vi "SQL查询.vi"(7 "condition":string, 8 "error in (no error)":errorcluster, 9 "columns":string[](array[string]), 10 "table输入":string(combo), 11 "database":string(combo)) -> (0 "error out":errorcluster, 1 "拆分数据":bool, 2 "columns输出":string[](array[string]), 3 "data":string[][](table))   [LabVIEW 2016, in "数据传输系统-04.lvlib"]
uses:
  <vilib>/Utility/sysdir.llb/System Directory Type.ctl
  <vilib>/addons/database/Connection.llb/DB Tools Open Connec (String).vi
  <vilib>/addons/database/_DB Variant To Data/Database Variant To Data.xnode
  <vilib>/addons/database/NI_Database_API.lvlib
panel:
  out "元素":string
  out "子数组":string[](array[string])
  # "时间 > #2021/01/15 08:00:00#and 时间 < #2021/04/15 08:00:00# order by 时间 asc"
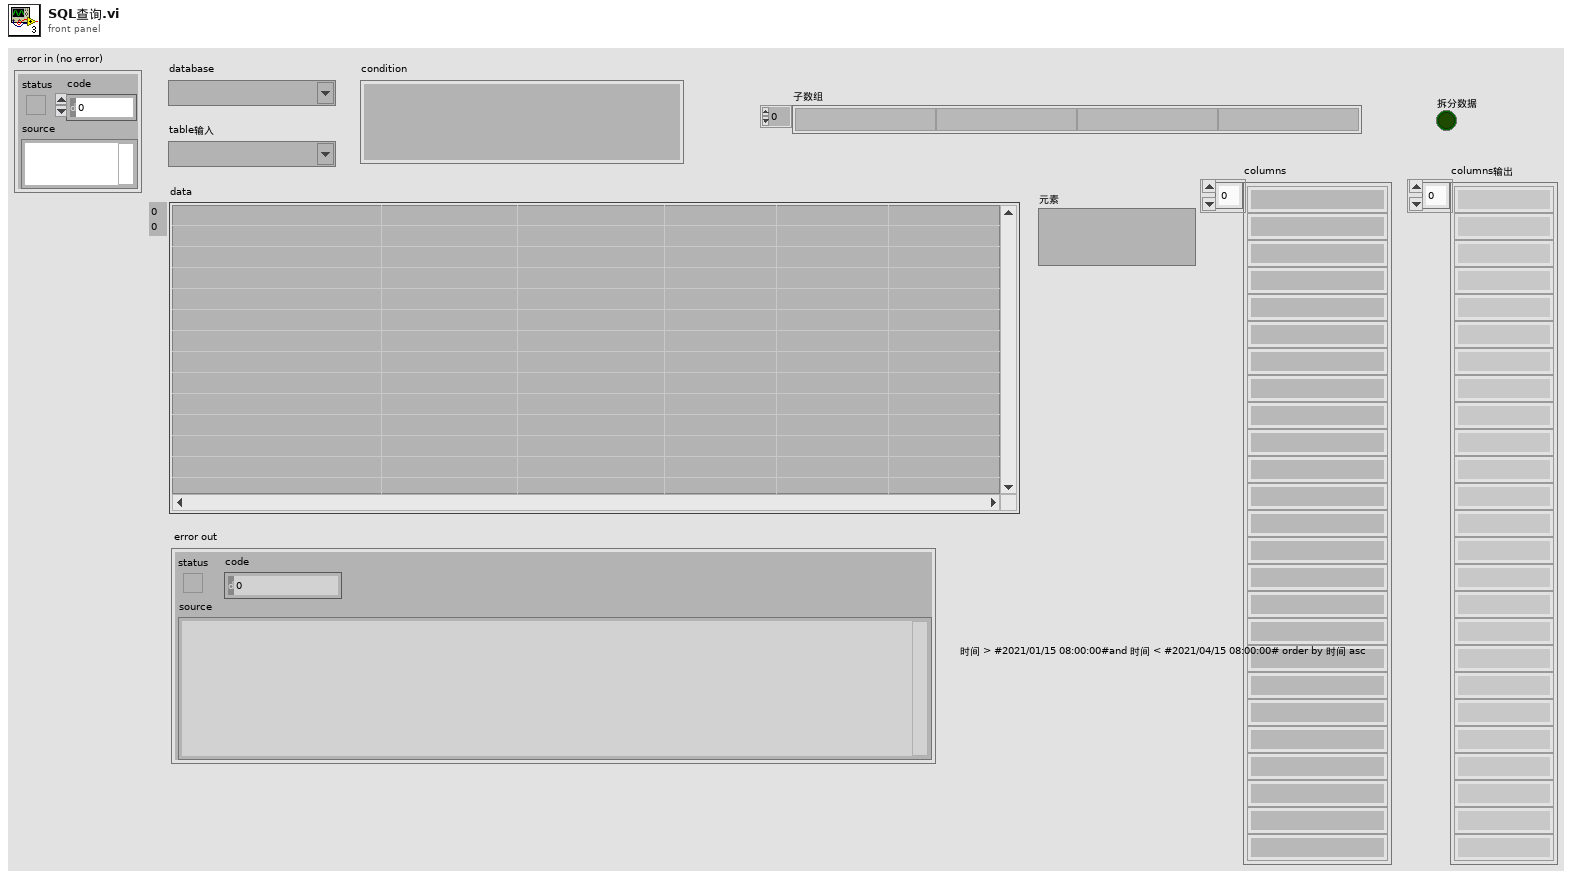
[diagram p1: front panel]
types:
  T1 = typedef "System Directory Type.ctl" = i32
  T2 = typedef "NI_Database_API.lvlib/Conn ObjectReference.ctl" = refnum<k1>
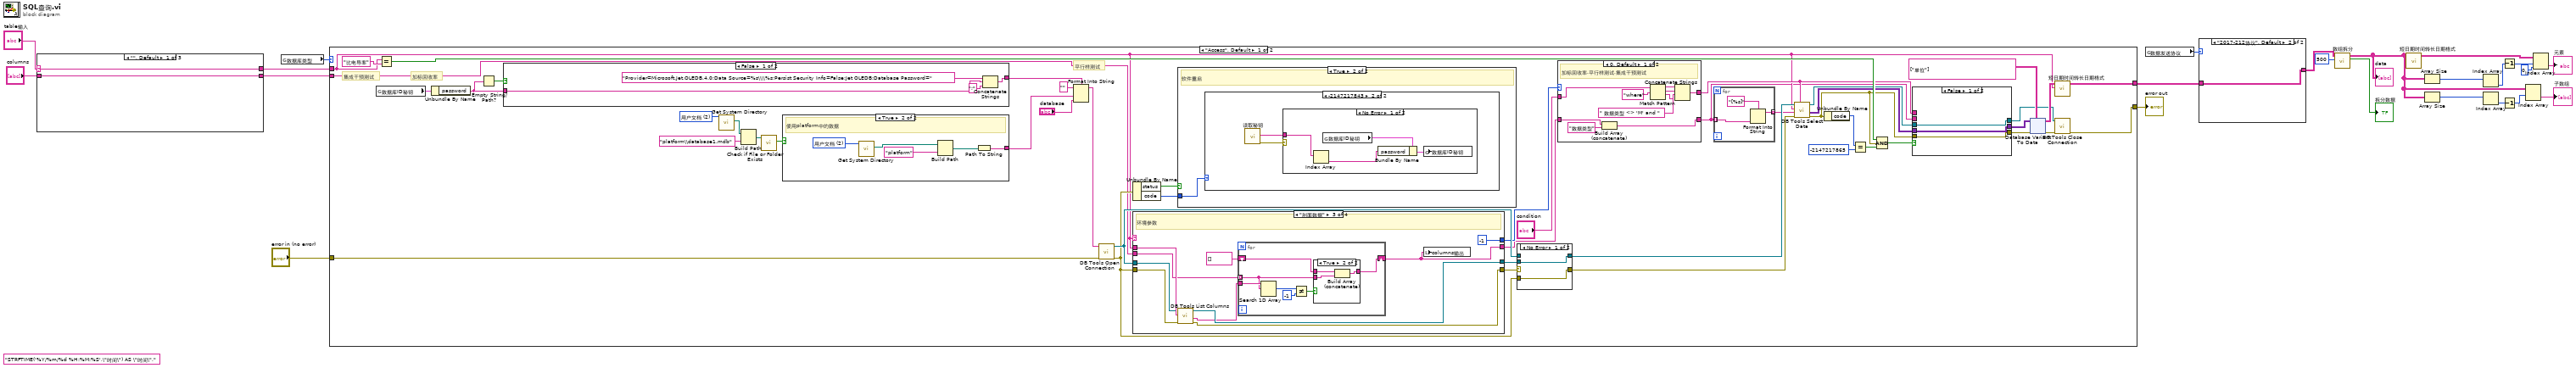
[diagram p0: block diagram]
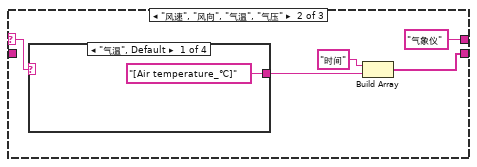
[diagram p2: hidden frame]
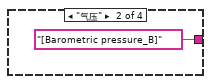
[diagram p3: hidden frame]
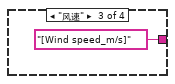
[diagram p4: hidden frame]
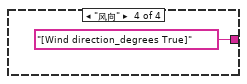
[diagram p5: hidden frame]
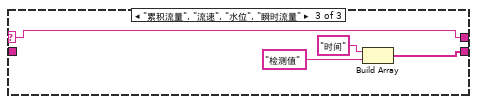
[diagram p6: hidden frame]
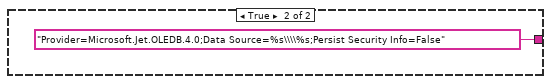
[diagram p7: hidden frame]
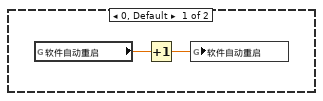
[diagram p9: hidden frame]
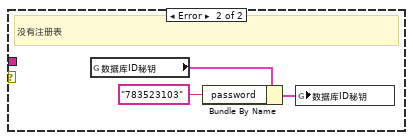
[diagram p10: hidden frame]
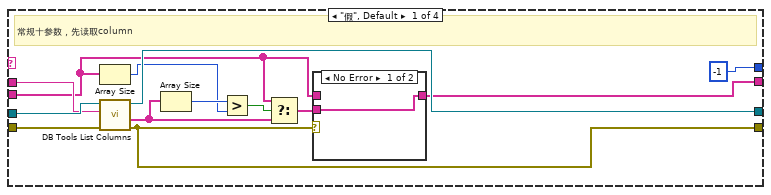
[diagram p13: hidden frame]
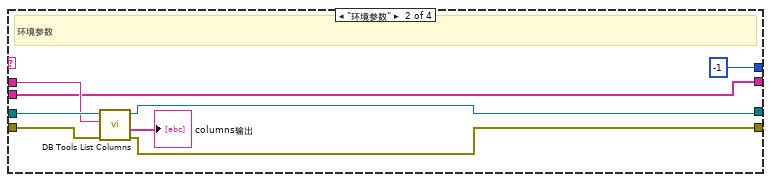
[diagram p15: hidden frame]
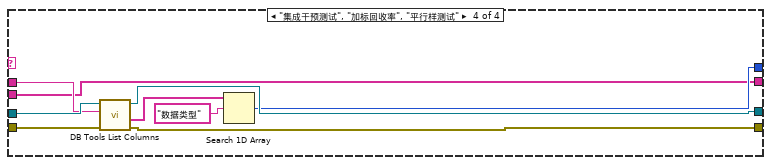
[diagram p17: hidden frame]
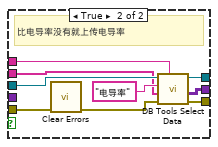
[diagram p18: hidden frame]
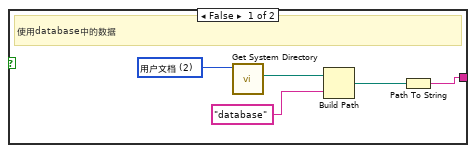
[diagram p19: hidden frame]
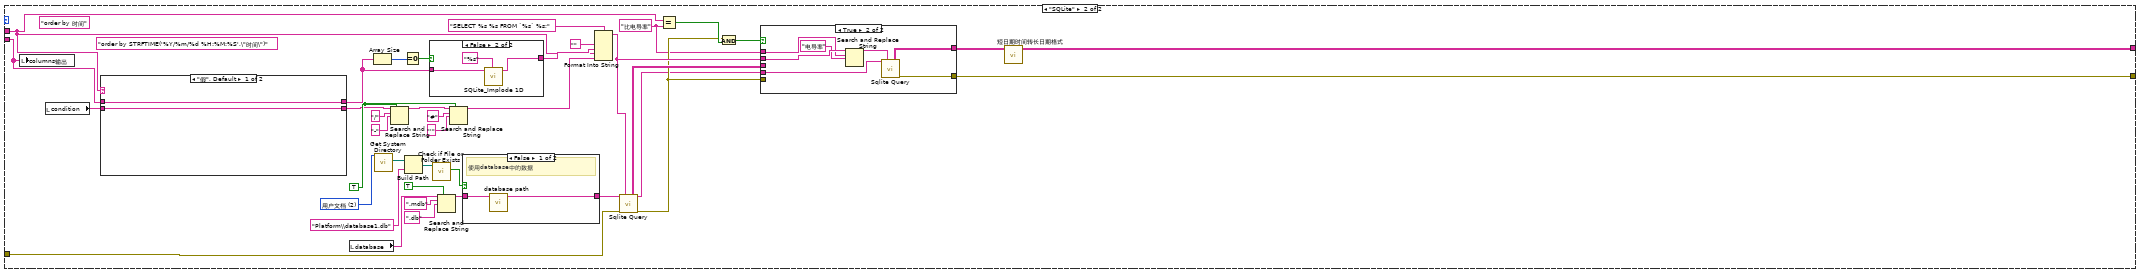
[diagram p20: hidden frame]
diagram:
  (unwired) "STRFTIME('%Y/%m/%d %H:%M:%S',\"时间\") AS \"时间\"," ("输入 1")
  n1 = case shown="\"\", Default" "table输入" {
    selector: "table输入" -> [w25 w29 w35]
    tunnel: [w25 "气象仪" w35] -> w4
    tunnel: "columns" -> [w24 _ _]
    tunnel: [w24 w26 w37] -> w5
    frame "", Default {
    }
    frame "风速", "风向", "气温", "气压" {
      n2 = case shown="\"气温\", Default" w29 {
        tunnel: ["[Air temperature_℃]" "[Barometric pressure_B]" "[Wind speed_m/s]" "[Wind direction_degrees True]"] -> w27
        frame "气温", Default {
        }
        frame "气压" {
        }
        frame "风速" {
        }
        frame "风向" {
        }
      }
      n3 = Build Array("时间", w27) -> (w26:string[])
    }
    frame "累积流量", "流速", "水位", "瞬时流量" {
      n4 = Build Array("时间", "检测值") -> (w37:string[])
    }
  }
  n5 = global read "断电保存全局.vi" "数据库类型"() -> (w8:enum16{"Access", "SQLite"})
  n6 = case shown="\"Access\", Default" w8 {
    tunnel: [w80 w274] -> w23
    tunnel: [w52 w250] -> w11
    tunnel: "error in (no error)" -> [w45 w243]
    tunnel: w5 -> [w43 w246]
    tunnel: w4 -> [w42 w245]
    frame "Access", Default {
      w78 = T1 2 items=["用户目录"=0, "用户桌面"=1, "用户文档"=2, "用户应用程序数据"=3, "用户设置"=4, "用户临时目录"=5, "公共文档"=6, "公共应用程序数据"=7, "公共设置"=8, "公共缓存"=13, "系统核心库"=9, "系统安装库"=10, "应用程序文件"=11, "启动盘根目录"=12] ("system directory type")
      # "集成干预测试"
      # "平行样测试"
      # "加标回收率"
      n7 = global read "外部交互全局.vi" "数据库ID秘钥"() -> (w46:cluster{"userID":string, "password":string})
      n8 = Equal?(x=w42, y="比电导率") -> (x = y?=w72:bool)
      n9 = Unbundle By Name(w46) -> ("password"=w47:string)
      n10 = Empty String/Path?(string/path=w47) -> (empty?=w49:bool)
      n11 = case shown="False" w49 {
        tunnel: [w89 "Provider=Microsoft.Jet.OLEDB.4.0;Data Source=%s\\\\%s;Persist Security Info=False" ("格式字符串")] -> w48
        tunnel: w47 -> [w92 _]
        frame False {
          n12 = Concatenate Strings("Provider=Microsoft.Jet.OLEDB.4.0;Data Source=%s\\\\%s;Persist Security Info=False;Jet OLEDB:Database Password=" ("格式字符串"), w92, ";" ("字符串")) -> (w89:string)
        }
        frame True {
        }
      }
      n13 = call <vilib>:"Get System Directory.vi"("system directory type"=w78) -> ("system directory"=w79:path)  [unwired: 10 in]
      n14 = Build Path(base path=w79, name or relative path="platform\\database1.mdb" ("condition")) -> (appended path=w77:path)
      n15 = call <vilib>:"Check if File or Folder Exists.vi"("path"=w77) -> ("file or folder exists?"=w75:bool)  [unwired: 8 in, 2 out]
      n16 = case shown="True" w75 {
        tunnel: [w187 w192] -> w74
        frame False {
          w190 = T1 2 items=["用户目录"=0, "用户桌面"=1, "用户文档"=2, "用户应用程序数据"=3, "用户设置"=4, "用户临时目录"=5, "公共文档"=6, "公共应用程序数据"=7, "公共设置"=8, "公共缓存"=13, "系统核心库"=9, "系统安装库"=10, "应用程序文件"=11, "启动盘根目录"=12] ("system directory type")
          # "使用database中的数据"
          n17 = call <vilib>:"Get System Directory.vi"("system directory type"=w190) -> ("system directory"=w189:path)  [unwired: 10 in]
          n18 = Build Path(base path=w189, name or relative path="database" ("condition")) -> (appended path=w191:path)
          n19 = Path To String(path=w191) -> (string=w187:string)
        }
        frame True {
          w196 = T1 2 items=["用户目录"=0, "用户桌面"=1, "用户文档"=2, "用户应用程序数据"=3, "用户设置"=4, "用户临时目录"=5, "公共文档"=6, "公共应用程序数据"=7, "公共设置"=8, "公共缓存"=13, "系统核心库"=9, "系统安装库"=10, "应用程序文件"=11, "启动盘根目录"=12] ("system directory type")
          # "使用platform中的数据"
          n20 = call <vilib>:"Get System Directory.vi"("system directory type"=w196) -> ("system directory"=w195:path)  [unwired: 10 in]
          n21 = Build Path(base path=w195, name or relative path="platform" ("condition")) -> (appended path=w193:path)
          n22 = Path To String(path=w193) -> (string=w192:string)
        }
      }
      n23 = Format Into String(format string=w48, initial string="" ("初始字符串"), w74, "database") -> (resulting string=w82:string)  [unwired: 1 in, 1 out]
      n24 = call-poly <vilib>:"DB Tools Open Connection.vi"("error in (no error)"=w45, "connection information"=w82) -> ("error out"=w53:errorcluster, "connection reference"=w58:T2)  [unwired: 6 in]
      n25 = Unbundle By Name(w53) -> ("status"=w51:bool, "code"=w41:i32)
      n26 = case shown="\"剖面数据\"" w42 {
        tunnel: w58 -> [w133 w144 w152 w174]
        tunnel: w53 -> [w130 w143 w151 w172]
        tunnel: [w131 w142 w149 w171] -> w60
        tunnel: [w125 w141 w150 w170] -> w61
        tunnel: w42 -> [w132 w140 w153 w173]
        tunnel: [-1 ("index of element") -1 ("index of element") -1 ("index of element") w167] -> w56
        tunnel: w43 -> [w122 w137 w148 w166]
        tunnel: [w123 w137 w145 w166] -> w54
        frame "假", Default {
          # "常规十参数，先读取column"
          n27 = Array Size(array=w122) -> (size(s)=w127:i32)
          n28 = call <vilib>:"DB Tools List Columns.vi"("error in (no error)"=w130, "table"=w132, "connection reference"=w133) -> ("error out"=w125:errorcluster, "columns"=w126:string[], "connection reference out"=w131:T2)  [unwired: 1 in, 1 out]
          n29 = Array Size(array=w126) -> (size(s)=w128:i32)
          n30 = Greater?(x=w128, y=w127) -> (0:w129:bool)
          n31 = Select(t=w122, s=w129, f=w126) -> (s? t:f=w124:string[])
          n32 = case shown="No Error" w125 {
            tunnel: w124 -> [w135 _]
            tunnel: [w135 w136] -> w123
            tunnel: w122 -> [_ w136]
            frame No Error {
            }
            frame Error {
            }
          }
        }
        frame "环境参数" {
          # "环境参数"
          n33 = call <vilib>:"DB Tools List Columns.vi"("error in (no error)"=w143, "table"=w140, "connection reference"=w144) -> ("error out"=w141:errorcluster, "columns"=→"columns输出":string[], "connection reference out"=w142:T2)  [unwired: 1 in, 1 out]
        }
        frame "剖面数据" {
          # "环境参数"
          n34 = call <vilib>:"DB Tools List Columns.vi"("error in (no error)"=w151, "table"=w153, "connection reference"=w152) -> ("error out"=w150:errorcluster, "columns"=w147:string[], "connection reference out"=w149:T2)  [unwired: 1 in, 1 out]
          n35 = for {
            tunnel: w148 -> [w157] mode=indexing
            tunnel: w147 -> [w161]
            shift-right: [w155] -> w145
            shift-left: string[] [] -> [w158]
            n36 = Search 1D Array(1D array=w161, element=w157) -> (index of element=w160:i32)  [unwired: 1 in]
            n37 = Not Equal?(x=w160, y=-1) -> (x != y?=w156:bool)
            n38 = case shown="True" w156 {
              tunnel: w158 -> [w162 w165]
              tunnel: w157 -> [_ w164]
              tunnel: [w162 w163] -> w155
              frame False {
              }
              frame True {
                n39 = Build Array (concatenate)(w165, w164) -> (w163:string[])
              }
            }
          }
          n40 = local write "columns输出"(w145) -> ()
        }
        frame "集成干预测试", "加标回收率", "平行样测试" {
          n41 = call <vilib>:"DB Tools List Columns.vi"("error in (no error)"=w172, "table"=w173, "connection reference"=w174) -> ("error out"=w170:errorcluster, "columns"=w169:string[], "connection reference out"=w171:T2)  [unwired: 1 in, 1 out]
          n42 = Search 1D Array(1D array=w169, element="数据类型" ("元素")) -> (index of element=w167:i32)  [unwired: 1 in]
        }
      }
      n43 = case shown="True" w51 {
        tunnel: w41 -> [_ w94]
        frame False {
        }
        frame True {
          # "软件重启"
          n44 = case shown="-2147217843" w94 {
            frame 0, Default {
              n45 = global read "全局1.vi" "软件自动重启"() -> (w96:dbl)
              n46 = Increment(x=w96) -> (x+1=w95:dbl)
              n47 = global write "全局1.vi" "软件自动重启"(w95) -> ()
            }
            frame -2147217843 {
              n48 = call "读取秘钥.vi"() -> ("error out"=w97:errorcluster, "值"=w98:string[])  [unwired: 9 in, 1 out]
              n49 = case shown="No Error" w97 {
                tunnel: w98 -> [w102 _]
                frame No Error {
                  n50 = Index Array(array=w102) -> (element=w99:string)  [unwired: 1 in]
                  n51 = global read "外部交互全局.vi" "数据库ID秘钥"() -> (w100:cluster{"userID":string, "password":string})
                  n52 = Bundle By Name(cluster=w100, "password"=w99) -> (w101:cluster{"userID":string, "password":string})
                  n53 = global write "外部交互全局.vi" "数据库ID秘钥"(w101) -> ()
                }
                frame Error {
                  # "没有注册表"
                  n54 = global read "外部交互全局.vi" "数据库ID秘钥"() -> (w104:cluster{"userID":string, "password":string})
                  n55 = Bundle By Name(cluster=w104, "password"="783523103") -> (w105:cluster{"userID":string, "password":string})
                  n56 = global write "外部交互全局.vi" "数据库ID秘钥"(w105) -> ()
                }
              }
            }
          }
        }
      }
      n57 = case shown="No Error" w61 {
        selector: w61 -> [_ w121]
        tunnel: w60 -> [w119 _]
        tunnel: [w119 w120] -> w59
        tunnel: w58 -> [_ w120]
        tunnel: [w118 w121] -> w57
        tunnel: w53 -> [w118 _]
        frame No Error {
        }
        frame Error {
        }
      }
      n58 = case "条件结构" shown="0, Default" w56 {
        tunnel: "condition" -> [w113 w116]
        tunnel: w54 -> [w115 w117]
        tunnel: [w107 w117] -> w40
        tunnel: [w106 w116] -> w50
        frame 0, Default {
          # "加标回收率,平行样测试,集成干预测试"
          n59 = Build Array (concatenate)(w115, "数据类型" ("元素")) -> (w107:string[])
          n60 = Match Pattern(string=w113, regular expression="where" ("正则表达式")) -> (before substring=w111:string, match substring=w110:string, after substring=w108:string)  [unwired: 1 in, 1 out]
          n61 = Concatenate Strings(w111, w110, " 数据类型 <> 'M' and " ("字符串"), w108) -> (w106:string)
        }
        frame -1 {
        }
      }
      n62 = for {
        tunnel: w40 -> [w88] mode=indexing
        tunnel: [w87] -> w39 mode=indexing
        n63 = Format Into String(format string="[%s]" ("格式字符串"), w88) -> (resulting string=w87:string)  [unwired: 2 in, 1 out]
      }
      n64 = call <vilib>:"DB Tools Select Data.vi"("condition"=w50, "error in (no error)"=w57, "columns"=w39, "table"=w42, "connection reference"=w59) -> ("error out"=w65:errorcluster, "data"=w67:variant[][], "connection reference out"=w70:T2)  [unwired: 1 in]
      n65 = Unbundle By Name(w65) -> ("code"=w64:i32)
      n66 = Equal?(x=w64, y=-2147217865 ("code")) -> (x = y?=w62:bool)
      n67 = Compound Arithmetic op=AND ("复合运算")(w72, w65, w62) -> (w71:bool)
      n68 = case shown="False" w71 {
        tunnel: w50 -> [_ w186]
        tunnel: w70 -> [w177 w185]
        tunnel: [w177 w180] -> w69
        tunnel: [w176 w181] -> w68
        tunnel: w67 -> [w176 _]
        tunnel: w65 -> [w175 w183]
        tunnel: [w175 w179] -> w66
        tunnel: w40 -> [_ w178]
        frame False {
        }
        frame True {
          # "比电导率没有就上传电导率"
          n69 = call <vilib>:"Clear Errors.vi"("error in (no error)"=w183) -> ("error out"=w182:errorcluster)  [unwired: 5 in, 1 out]
          n70 = call <vilib>:"DB Tools Select Data.vi"("condition"=w186, "error in (no error)"=w182, "columns"=w178, "table"="电导率", "connection reference"=w185) -> ("error out"=w179:errorcluster, "data"=w181:variant[][], "connection reference out"=w180:T2)  [unwired: 1 in]
        }
      }
      n71 = xnode "Database Variant To Data"("database variant"=w68, "error in (no error)"=w66, "type"=string[][] [["单位"]]) -> ("data"=w81:string[][], "error out"=w83:errorcluster)
      n72 = call "短日期时间转长日期格式.vi"("table输入"=w42, "data"=w81) -> ("输出数组"=w80:string[][])  [unwired: 9 in]
      n73 = call <vilib>:"DB Tools Close Connection.vi"("error in (no error)"=w83, "connection reference"=w69) -> ("error out"=w52:errorcluster)  [unwired: 5 in]
    }
    frame "SQLite" {
      w248 = "比电导率" ("y")
      (unwired) "order by STRFTIME('%Y/%m/%d %H:%M:%S',\"时间\")" ("替换字符串(\"\")")
      (unwired) "order by 时间" ("搜索字符串")
      w259 = TRUE ("替换全部？(F)")
      w276 = T1 2 items=["用户目录"=0, "用户桌面"=1, "用户文档"=2, "用户应用程序数据"=3, "用户设置"=4, "用户临时目录"=5, "公共文档"=6, "公共应用程序数据"=7, "公共设置"=8, "公共缓存"=13, "系统核心库"=9, "系统安装库"=10, "应用程序文件"=11, "启动盘根目录"=12] ("system directory type")
      n74 = local write "columns输出"(w246) -> ()
      n75 = local read "condition"() -> (w258:string)
      n76 = case shown="\"假\", Default" w245 {
        tunnel: w258 -> [w290 w296]
        tunnel: w246 -> [w289 w298]
        tunnel: [w289 w297] -> w269
        tunnel: [w290 w295] -> w257
        frame "假", Default {
        }
        frame "集成干预测试", "加标回收率", "平行样测试" {
          n77 = Build Array (concatenate)(w298, "数据类型" ("元素")) -> (w297:string[])
          n78 = call "数据库加密匹配 (子VI).vi"("输入参数"="N") -> ("Encoded String"=w293:string)  [unwired: 10 in]
          n79 = Match Pattern(string=w296, regular expression="where" ("正则表达式")) -> (before substring=w301:string, match substring=w300:string, after substring=w299:string)  [unwired: 1 in, 1 out]
          n80 = Format Into String(format string=" 数据类型 = '%s' and " ("字符串"), w293) -> (resulting string=w291:string)  [unwired: 2 in, 1 out]
          n81 = Concatenate Strings(w301, w300, w291, w299) -> (w295:string)
        }
      }
      n82 = local read "database"() -> (w261:string)
      n83 = Array Size(array=w269) -> (size(s)=w273:i32)
      n84 = call <vilib>:"Get System Directory.vi"("system directory type"=w276) -> ("system directory"=w275:path)  [unwired: 10 in]
      n85 = Search and Replace String(replace all?=w259, input string=w257, search string="/" ("搜索字符串"), replace string="-" ("替换字符串(\"\")")) -> (result string=w266:string)  [unwired: 4 in, 3 out]
      n86 = Equal To 0?(x=w273) -> (x = 0?=w272:bool)
      n87 = Build Path(base path=w275, name or relative path="Platform\\database1.db" ("condition")) -> (appended path=w277:path)
      n88 = case shown="False" w272 {
        tunnel: w269 -> [_ w306]
        tunnel: ["*" ("t") w305] -> w270
        frame True {
        }
        frame False {
          n89 = call <userlib>:"SQLite_Implode 1D.vi"("Values"=w306, "format string"="%s") -> ("imploded string"=w305:string)  [unwired: 7 in, 1 out]
        }
      }
      n90 = call <vilib>:"Check if File or Folder Exists.vi"("path"=w277) -> ("file or folder exists?"=w279:bool)  [unwired: 8 in, 2 out]
      n91 = Search and Replace String(replace all?=TRUE ("替换全部？(F)"), input string=w261, search string=".mdb" ("搜索字符串"), replace string=".db" ("替换字符串(\"\")")) -> (result string=w256:string)  [unwired: 4 in, 3 out]
      n92 = Search and Replace String(replace all?=w259, input string=w266, search string="#" ("搜索字符串"), replace string="'" ("替换字符串(\"\")")) -> (result string=w241:string)  [unwired: 4 in, 3 out]
      n93 = case shown="False" w279 {
        tunnel: [w309 w310] -> w244
        tunnel: w256 -> [w308 w311]
        frame False {
          # "使用database中的数据"
          n94 = call "database path.vi"("database"=w308) -> ("Path out"=w309:string)  [unwired: 9 in, 1 out]
        }
        frame True {
          # "使用platform中的数据"
          n95 = call "database platform path.vi"("database"=w311) -> ("Path out"=w310:string)  [unwired: 10 in]
        }
      }
      n96 = Format Into String(format string="SELECT %s %s FROM `%s` %s;" ("SQL Query"), "", w270, w245, w241) -> (resulting string=w251:string)  [unwired: 2 in, 1 out]
      n97 = call "Sqlite Query.vi"("DB Path"=w244, "SQL Query"=w251, "error in (no error)"=w243) -> ("Results"=w253:string[][], "DB Path Out"=w247:string, "error out"=w249:errorcluster)  [unwired: 10 in]
      n98 = Equal?(x=w245, y=w248) -> (x = y?=w255:bool)
      n99 = And(x=w249, y=w255) -> (x .and. y?=w254:bool)
      n100 = case shown="True" w254 {
        tunnel: w253 -> [w281 _]
        tunnel: [w281 w288] -> w252
        tunnel: w251 -> [_ w285]
        tunnel: w247 -> [_ w287]
        tunnel: [w280 w286] -> w250
        tunnel: w249 -> [w280 _]
        tunnel: w248 -> [_ w284]
        frame False {
        }
        frame True {
          n101 = Search and Replace String(input string=w285, search string=w284, replace string="电导率" ("Tables Name")) -> (result string=w282:string)  [unwired: 5 in, 3 out]
          n102 = call "Sqlite Query.vi"("DB Path"=w287, "SQL Query"=w282) -> ("Results"=w288:string[][], "error out"=w286:errorcluster)  [unwired: 11 in, 1 out]
        }
      }
      n103 = call "短日期时间转长日期格式.vi"("data"=w252) -> ("输出数组"=w274:string[][])  [unwired: 10 in]
    }
  }
  "error out" <- w11
  n104 = global read "断电保存全局.vi" "数据发送协议"() -> (w22:enum16{"2005-212协议", "2017-212协议"})
  n105 = case shown="\"2017-212协议\", Default" w22 {
    tunnel: w23 -> [w313 w320]
    tunnel: [w312 w320] -> w9
    frame "2005-212协议" {
      n106 = for {
        N: 1 -> [_]
        tunnel: string[][] [] ("data") -> [w319]
        tunnel: w313 -> [w318] mode=indexing
        tunnel: [w316] -> w312
        n107 = Insert Into Array(array=w319, index (row)=0 ("索引 (行)"), new element=w318) -> (w316:string[][])  [unwired: 1 in]
      }
    }
    frame "2017-212协议", Default {
    }
  }
  n108 = call "数组拆分.vi"("拆分大小"=500, "输入数据"=w9) -> ("拆分数据"=→"拆分数据":bool, "输出数组"=w1:string[][])  [unwired: 8 in]
  "data" <- w1
  n109 = call "短日期时间转长日期格式.vi"("data"=w1) -> ("输出数组"=w17:string[][])  [unwired: 10 in]
  n110 = Array Size(array=w1) -> (size(s)=w16:i32[])
  n111 = Array Size(array=w1) -> (size(s)=w21:i32[])
  n112 = Index Array(array=w16) -> (element=w15:i32)  [unwired: 1 in]
  n113 = Index Array(array=w21) -> (element=w19:i32)  [unwired: 1 in]
  n114 = Decrement(x=w15) -> (x-1=w14:i32)
  n115 = Decrement(x=w19) -> (x-1=w18:i32)
  n116 = Index Array(array=w1, index (row)=w18) -> (element=→"子数组":string[])  [unwired: 1 in]
  n117 = Index Array(array=w17, index (row)=w14, index (col)=0 ("禁用的索引 (列)")) -> (element=→"元素":string)
